vi "monochromatorGetLastMessage.vi"(8 "error in":errorcluster, 11 "monochromator":refnum<k24>) -> (0 "error out":errorcluster, 2 "message":string, 3 "reference out":refnum<k24>)   [LabVIEW 2009]
doc: "Get last message generated by events and logged by the Cornerstonen driver/wrapper"
uses:
  C:/Users/anderson.chen/Desktop/Software Development/Cornerstone Series API (LV9)/Cornerstone DLL/Cornerstone.dll
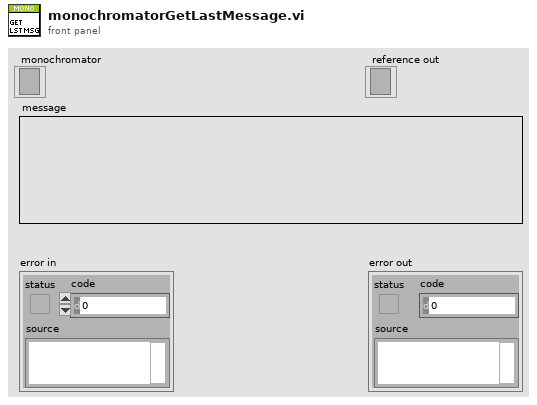
[diagram p1: front panel]
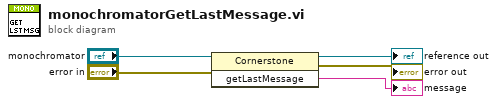
[diagram p0: block diagram]
diagram:
  n1 = invoke class="Cornerstone" method="getLastMessage"(reference="monochromator", error in="error in") -> (reference out=→"reference out":refnum<k24>, error out=→"error out":errorcluster, "getLastMessage"=→"message":string)  [unwired: 1 in]
